vi "Simple UDP Client.vi"() -> ()   [LabVIEW 2014, in "ESP8266 WiFi Wrapper.lvlib"]
uses:
  ESP8266 WiFi Wrapper.lvlib
  <vilib>/Aledyne-TSXperts/Arduino Compatible Compiler for LabVIEW/Arduino Compatible Compiler for LabVIEW.lvlib
panel:
  in  "Remote IP address":u8[](array[numeric])=[192, 168, 0, 47]
  in  "DNS address":u8[](array[numeric])=[0, 0, 0, 0]
  in  "IP address":u8[](array[numeric])=[192, 168, 0, 42]
  in  "Gateway":u8[](array[numeric])=[192, 168, 0, 1]
  in  "Subnet mask":u8[](array[numeric])=[255, 255, 255, 0]
  in  "Password":string="12345678"
  in  "SSID":string="ESP8266 Wifi UDP"
  in  "Listen Port":i16=8080
  in  "error in (no error)":errorcluster
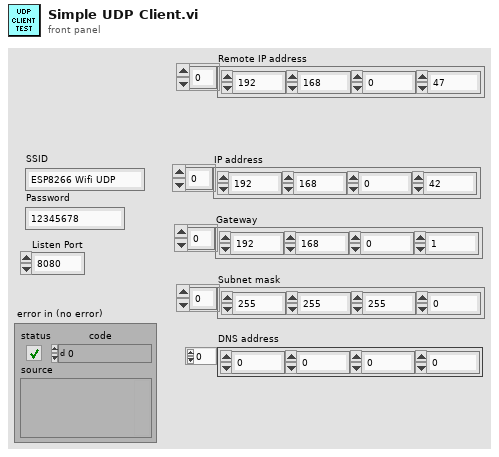
[diagram p1: front panel]
types:
  T1 = enum16{"WIFI_OFF", "WIFI_STA", "WIFI_AP", "WIFI_AP_STA"}
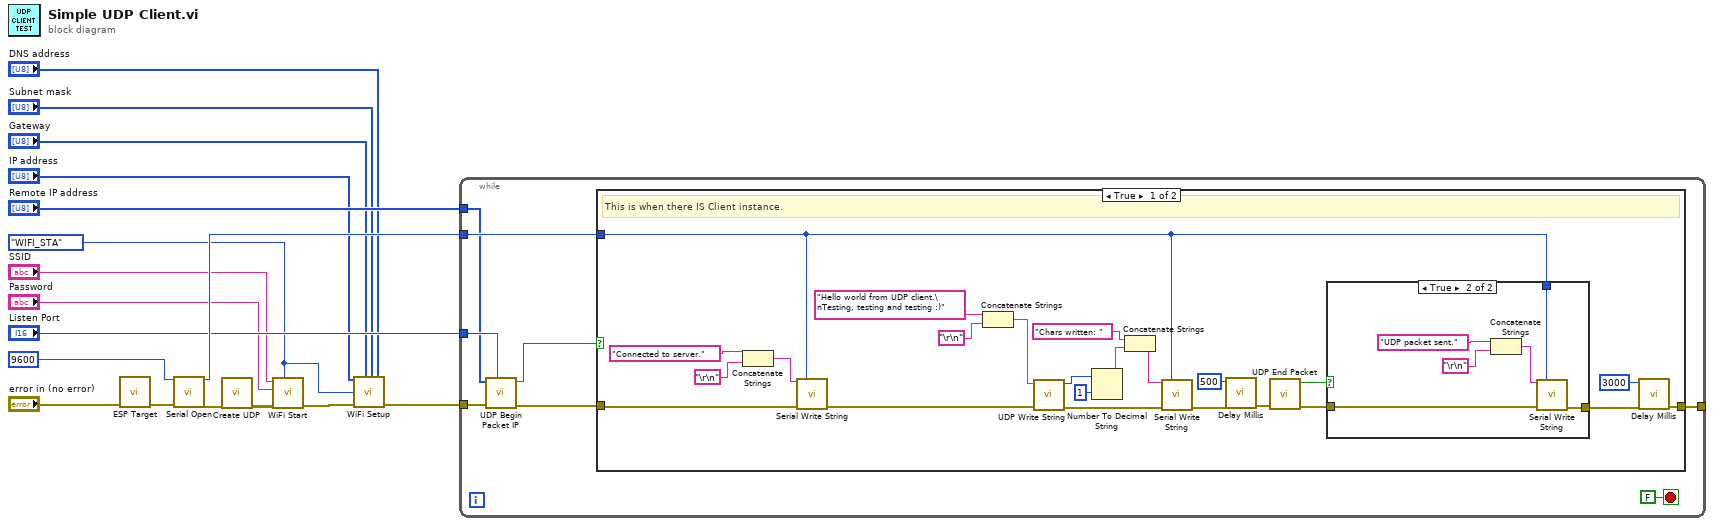
[diagram p0: block diagram]
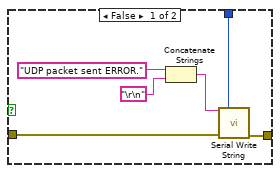
[diagram p2: hidden frame]
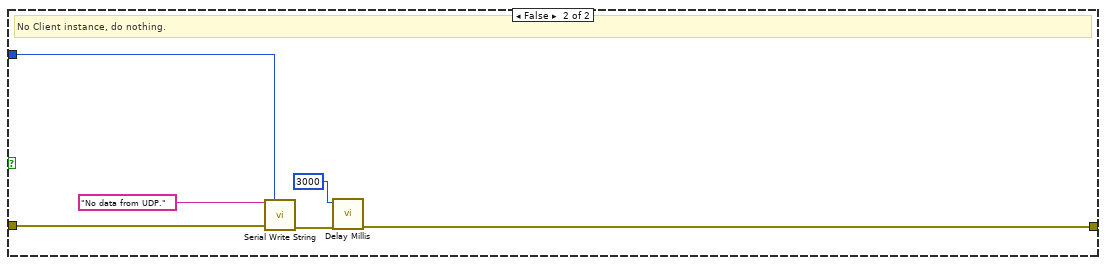
[diagram p3: hidden frame]
diagram:
  w1 = T1."WIFI_STA" ("WiFi Server Mode")
  n1 = call "ESP Target.vi"("Error In"="error in (no error)") -> ("Error Out"=w15:errorcluster)  [unwired: 10 in]
  n2 = call <vilib>:"Serial Open.vi"("Speed"=u32 9600, "error in (no error)"=w15) -> ("Instance"=w16:u8, "error out"=w11:errorcluster)  [unwired: 12 in]
  n3 = call "Create UDP.vi"("Error In"=w11) -> ("Error Out"=w10:errorcluster)  [unwired: 10 in]
  n4 = call "WiFi Start.vi"("WiFi Mode"=w1, "Error In"=w10, "Password"="Password", "SSID"="SSID") -> ("Error Out"=w3:errorcluster)  [unwired: 7 in]
  n5 = call "WiFi Setup.vi"("IP address"="IP address", "Gateway address"="Gateway", "Subnet mask"="Subnet mask", "DNS address"="DNS address", "WiFi Mode"=w1, "Error In"=w3) -> ("Error Out"=w2:errorcluster)  [unwired: 9 in]
  n6 = while {
    tunnel: w16 -> [w24]
    tunnel: [w23] -> _
    tunnel: w2 -> [w22]
    tunnel: "Listen Port" -> [w21]
    tunnel: "Remote IP address" -> [w18]
    stop <- FALSE stop-if-true
    n7 = call "UDP Begin Packet IP.vi"("Port"=w21, "Error In"=w22, "IP Address"=w18) -> ("Error Out"=w19:errorcluster, "Successful?"=w20:bool)  [unwired: 7 in]
    n8 = case shown="True" w20 {
      tunnel: w24 -> [w34 w65]
      tunnel: [w44 w62] -> w23
      tunnel: w19 -> [w39 w61]
      frame True {
        # "This is when there IS Client instance."
        n9 = Concatenate Strings("Connected to server." ("String"), "\r\n") -> (w46:string)
        n10 = call <vilib>:"Serial Write String.vi"("String"=w46, "Instance"=w34, "error in (no error)"=w39) -> ("error out"=w40:errorcluster)  [unwired: 12 in]
        n11 = Concatenate Strings("Hello world from UDP client.\nTesting, testing and testing :)" ("String"), "\r\n") -> (w36:string)
        n12 = call "UDP Write String.vi"("Error In"=w40, "String to write"=w36) -> ("Error Out"=w35:errorcluster, "Chars written"=w33:u8)  [unwired: 8 in]
        n13 = Number To Decimal String(number=w33, width (-)=i16 1) -> (decimal integer string=w31:string)
        n14 = Concatenate Strings("Chars written: " ("string"), w31) -> (w32:string)
        n15 = call <vilib>:"Serial Write String.vi"("String"=w32, "Instance"=w34, "error in (no error)"=w35) -> ("error out"=w28:errorcluster)  [unwired: 12 in]
        n16 = call <vilib>:"Delay Millis.vi"("error in (no error)"=w28, "delay"=u32 500) -> ("error out"=w29:errorcluster)  [unwired: 9 in]
        n17 = call "UDP End Packet.vi"("Error In"=w29) -> ("Error Out"=w43:errorcluster, "Successful?"=w42:bool)  [unwired: 9 in]
        n18 = case shown="True" w42 {
          tunnel: w43 -> [w51 w56]
          tunnel: w34 -> [w49 w57]
          tunnel: [w50 w55] -> w41
          frame False {
            n19 = Concatenate Strings("UDP packet sent ERROR." ("String"), "\r\n") -> (w52:string)
            n20 = call <vilib>:"Serial Write String.vi"("String"=w52, "Instance"=w49, "error in (no error)"=w51) -> ("error out"=w50:errorcluster)  [unwired: 12 in]
          }
          frame True {
            n21 = Concatenate Strings("UDP packet sent." ("String"), "\r\n") -> (w58:string)
            n22 = call <vilib>:"Serial Write String.vi"("String"=w58, "Instance"=w57, "error in (no error)"=w56) -> ("error out"=w55:errorcluster)  [unwired: 12 in]
          }
        }
        n23 = call <vilib>:"Delay Millis.vi"("error in (no error)"=w41, "delay"=u32 3000) -> ("error out"=w44:errorcluster)  [unwired: 9 in]
      }
      frame False {
        # "No Client instance, do nothing."
        n24 = call <vilib>:"Serial Write String.vi"("String"="No data from UDP.", "Instance"=w65, "error in (no error)"=w61) -> ("error out"=w64:errorcluster)  [unwired: 12 in]
        n25 = call <vilib>:"Delay Millis.vi"("error in (no error)"=w64, "delay"=u32 3000) -> ("error out"=w62:errorcluster)  [unwired: 9 in]
      }
    }
  }
